vi "Calibration-Frame12.vi"(6 "Din":dbl[](array[numeric]), 7 "Ein":dbl[](array[numeric]), 9 "CsortBy":dbl[](array[numeric]), 10 "Bin":dbl[](array[numeric]), 11 "Ain":dbl[](array[numeric])) -> (2 "ArrayCABDE":dbl[][](array[numeric]), 3 "Sort Index":i32[](array[numeric]))   [LabVIEW 2020]
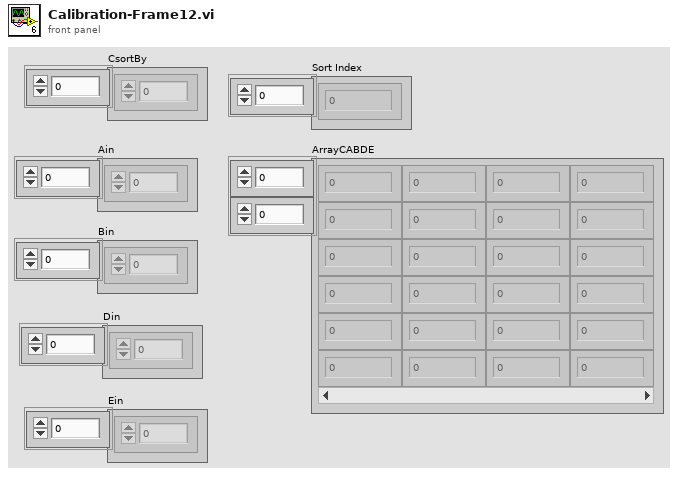
[diagram p1: front panel]
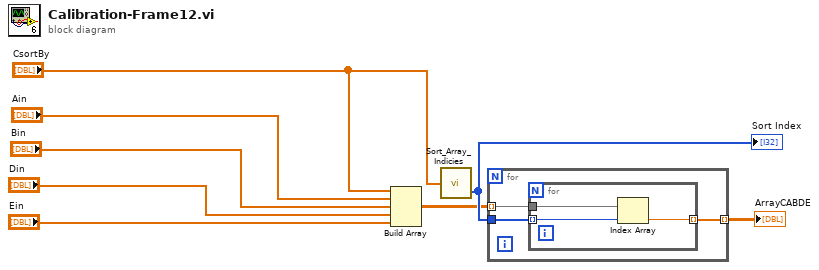
[diagram p0: block diagram]
diagram:
  n1 = Build Array("CsortBy", "Ain", "Bin", "Din", "Ein") -> (w5:dbl[][])
  n2 = call "Sort_Array_Indicies.vi"("unsorted array"="CsortBy") -> ("Sort Index"=w8:i32[])  [unwired: 1 out]
  "Sort Index" <- w8
  n3 = for {
    tunnel: w8 -> [w11]
    tunnel: w5 -> [w10] mode=indexing
    tunnel: [w9] -> w6 mode=indexing
    n4 = for {
      tunnel: w11 -> [w14] mode=indexing
      tunnel: w10 -> [w13]
      tunnel: [w12] -> w9 mode=indexing
      n5 = Index Array(array=w13, index=w14) -> (element=w12:dbl)
    }
  }
  "ArrayCABDE" <- w6
